vi "[CS] [Frame] Save to Image File.vi"(9 "image data":T1, 10 "Name":string, 11 "base path":path) -> ()   [LabVIEW 2014]
uses:
  <vilib>/picture/picture.llb/imagedata.ctl
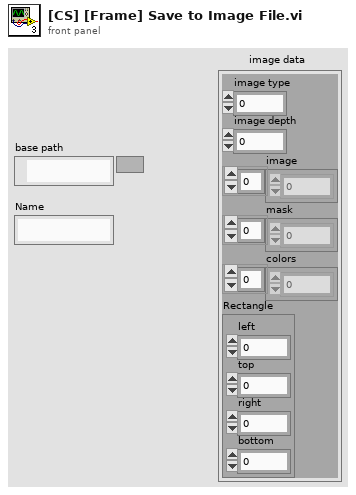
[diagram p1: front panel]
types:
  T1 = typedef "imagedata.ctl" = cluster{"image type":i32, "image depth":i32, "image":u8[], "mask":u8[], "colors":u32[], "Rectangle":cluster{"left":i16, "top":i16, "right":i16, "bottom":i16}}
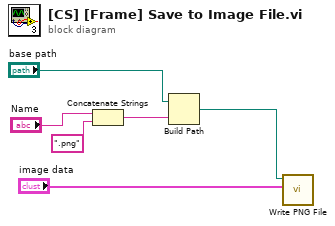
[diagram p0: block diagram]
diagram:
  n1 = Concatenate Strings("Name", ".png" ("string")) -> (w3:string)
  n2 = Build Path(base path="base path", name or relative path=w3) -> (appended path=w4:path)
  n3 = call <vilib>:"Write PNG File.vi"("image data"="image data", "path to PNG file"=w4) -> ()  [unwired: 8 in, 2 out]
